vi "Torque_Application_11.20.vi"() -> ()   [LabVIEW 2016]
uses:
  Desktop/Controls_Framework_Spring17_LV14_pwm_1_enc_2(1)/Controls_Framework_Spring17_LV14_pwm_1_enc_2/Controls_Framework_Spring17_LV14_pwm_1_enc_2/FGVsandTypeDefs/System Selection.ctl
  Desktop/Controls_Framework_Spring17_LV14_pwm_1_enc_2(1)/Controls_Framework_Spring17_LV14_pwm_1_enc_2/Controls_Framework_Spring17_LV14_pwm_1_enc_2/FGVsandTypeDefs/Data Out.ctl
  Desktop/Controls_Framework_Spring17_LV14_pwm_1_enc_2(1)/Controls_Framework_Spring17_LV14_pwm_1_enc_2/Controls_Framework_Spring17_LV14_pwm_1_enc_2/tools/digitalArrayTool.vi
  Desktop/Controls_Framework_Spring17_LV14_pwm_1_enc_2(1)/Controls_Framework_Spring17_LV14_pwm_1_enc_2/Controls_Framework_Spring17_LV14_pwm_1_enc_2/hardware/ootb/OOTB Write.vi
  Desktop/Controls_Framework_Spring17_LV14_pwm_1_enc_2(1)/Controls_Framework_Spring17_LV14_pwm_1_enc_2/Controls_Framework_Spring17_LV14_pwm_1_enc_2/hardware/sadi/SADI Write.vi
  Desktop/Controls_Framework_Spring17_LV14_pwm_1_enc_2(1)/Controls_Framework_Spring17_LV14_pwm_1_enc_2/Controls_Framework_Spring17_LV14_pwm_1_enc_2/FGVsandTypeDefs/FGV System.vi
  <vilib>/Utility/semaphor.llb/Acquire Semaphore.vi
  Desktop/Controls_Framework_Spring17_LV14_pwm_1_enc_2(1)/Controls_Framework_Spring17_LV14_pwm_1_enc_2/Controls_Framework_Spring17_LV14_pwm_1_enc_2/hardware/simulations/MotorSimulation/SingleMotorSystem-HbridgeSimple-DAQ.vi
  Desktop/Controls_Framework_Spring17_LV14_pwm_1_enc_2(1)/Controls_Framework_Spring17_LV14_pwm_1_enc_2/Controls_Framework_Spring17_LV14_pwm_1_enc_2/hardware/simulations/MotorSimulation/DoubleMotorSystem-HbridgeTurnOn-DAQ.vi
  Desktop/Controls_Framework_Spring17_LV14_pwm_1_enc_2(1)/Controls_Framework_Spring17_LV14_pwm_1_enc_2/Controls_Framework_Spring17_LV14_pwm_1_enc_2/hardware/simulations/FurutaPendulum/FurutaPendulumSystem-HbridgeSimple-DAQ.vi
  <vilib>/Utility/semaphor.llb/Release Semaphore.vi
  Desktop/Controls_Framework_Spring17_LV14_pwm_1_enc_2(1)/Controls_Framework_Spring17_LV14_pwm_1_enc_2/Controls_Framework_Spring17_LV14_pwm_1_enc_2/hardware/ootb/OOTB Slowdown.vi
  Desktop/Controls_Framework_Spring17_LV14_pwm_1_enc_2(1)/Controls_Framework_Spring17_LV14_pwm_1_enc_2/Controls_Framework_Spring17_LV14_pwm_1_enc_2/hardware/ootb/OOTB Stop.vi
  Desktop/Controls_Framework_Spring17_LV14_pwm_1_enc_2(1)/Controls_Framework_Spring17_LV14_pwm_1_enc_2/Controls_Framework_Spring17_LV14_pwm_1_enc_2/hardware/sadi/SADI Slowdown.vi
  Desktop/Controls_Framework_Spring17_LV14_pwm_1_enc_2(1)/Controls_Framework_Spring17_LV14_pwm_1_enc_2/Controls_Framework_Spring17_LV14_pwm_1_enc_2/hardware/sadi/SADI Stop.vi
  <vilib>/Utility/semaphor.llb/Release Semaphore Reference.vi
panel:
  out "Numeric 3":i32=10818974
  out "AI0 3":dbl=2.506715973370057
  out "Torque End 2":dbl=964.1691552387538
  in  "+ Torque":dbl=100.0 format="%#_13g"
  in  "- Torque":dbl=-100.0 format="%#_13g"
  out "Torque 3":dbl=964.1691552387538
  out "AI Graph 3":dbl(graph)
  out "Torque 2":dbl=1035.2691658522822
  out "AI Graph 2":dbl(graph)
  out "Torque 1":dbl=964.1691552387538
  out "AI Graph 1":dbl(graph)
  out "Numeric":i32=10818974
  out "AI0":dbl=2.506715973370057
  out "Torque Before":dbl=964.1691552387538
  out "savedSections 2":u32 caption="# Sections Saved"
  out "saveTime 2":dbl caption="Total Save Time (s)" format="%#.3g"
  in  "Stop?":bool
  in  "Save?":bool
  in  "System":T1=enum."SADI DAQ"
  in  "Controller?":bool
  in  "AO Voltages [V]":cluster{"AO0":dbl, "AO1":dbl} {"AO1" min=0.0 max=5.0 step=0.01; "AO0" min=0.0 max=5.0 step=0.01}
  out "AI Voltages [V]":T2={"AI0"=2.4857487004494705, "AI1"=0.0018539516886717992, "AI2"=-0.01062114806262072, "AI3"=0.020274310509003104, "ENC0"=0, "ENC1"=0}
  in  "Tab Control":T3(tab)
  out "AI Graph":T4(graph)={"AI0"=2.4857487004494705, "AI1"=0.0018539516886717992, "AI2"=-0.01062114806262072, "AI3"=0.020274310509003104, "ENC0"=0, "ENC1"=0}
  # "Many of these controls are locked. Do not copy them.\nPlace a new control by right clicking anywhere in the front panel."
  # "v4.3.1"
  # "Time Information"
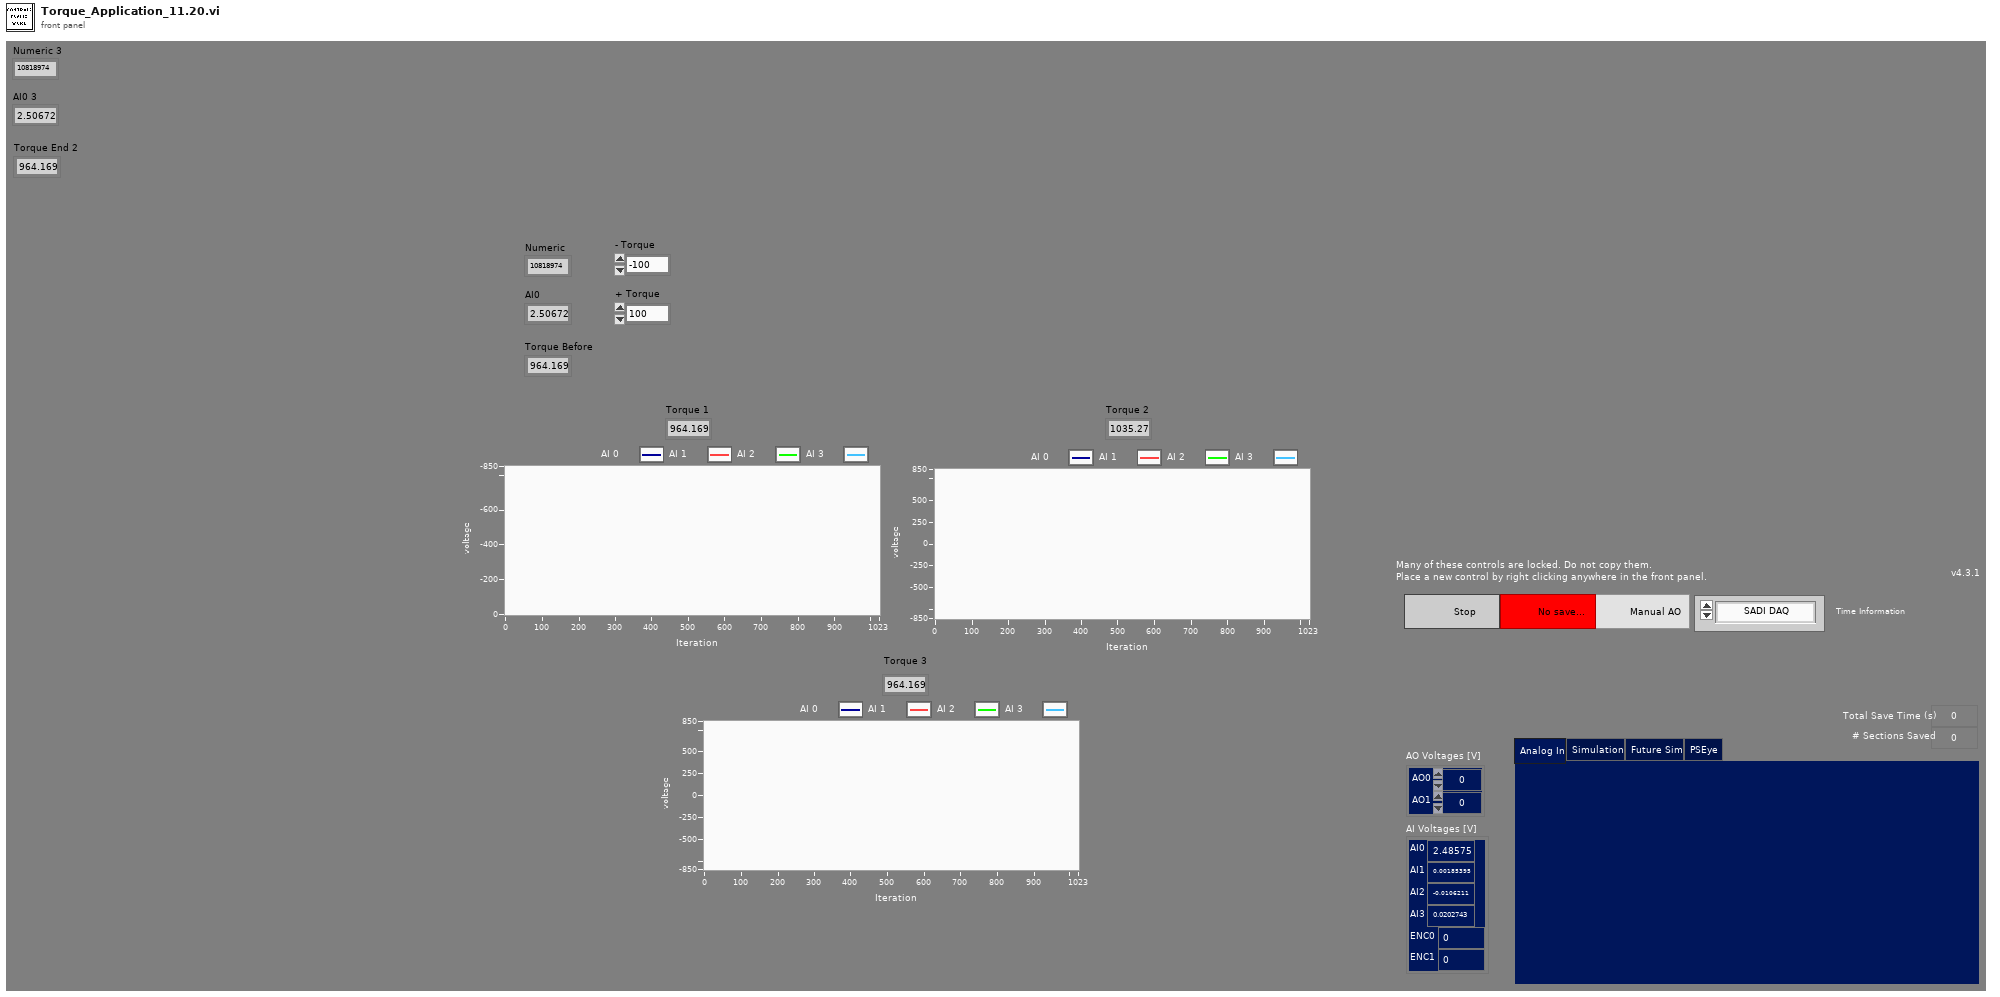
[diagram p1: front panel]
types:
  T1 = typedef "System Selection.ctl" = enum16{"OOTB DAQ", "SADI DAQ", "Single Motor Simulation", "Double Motor Simulation", "Furuta Pendulum"}
  T2 = typedef "Data Out.ctl" = cluster{"AI0":dbl, "AI1":dbl, "AI2":dbl, "AI3":dbl, "ENC0":i32, "ENC1":i32}
  T3 = enum32{"Analog In", "Simulation", "Future Sim", "PSEye"}
  T4 = cluster{"AI0":dbl, "AI1":dbl, "AI2":dbl, "AI3":dbl, "ENC0":i32, "ENC1":i32}
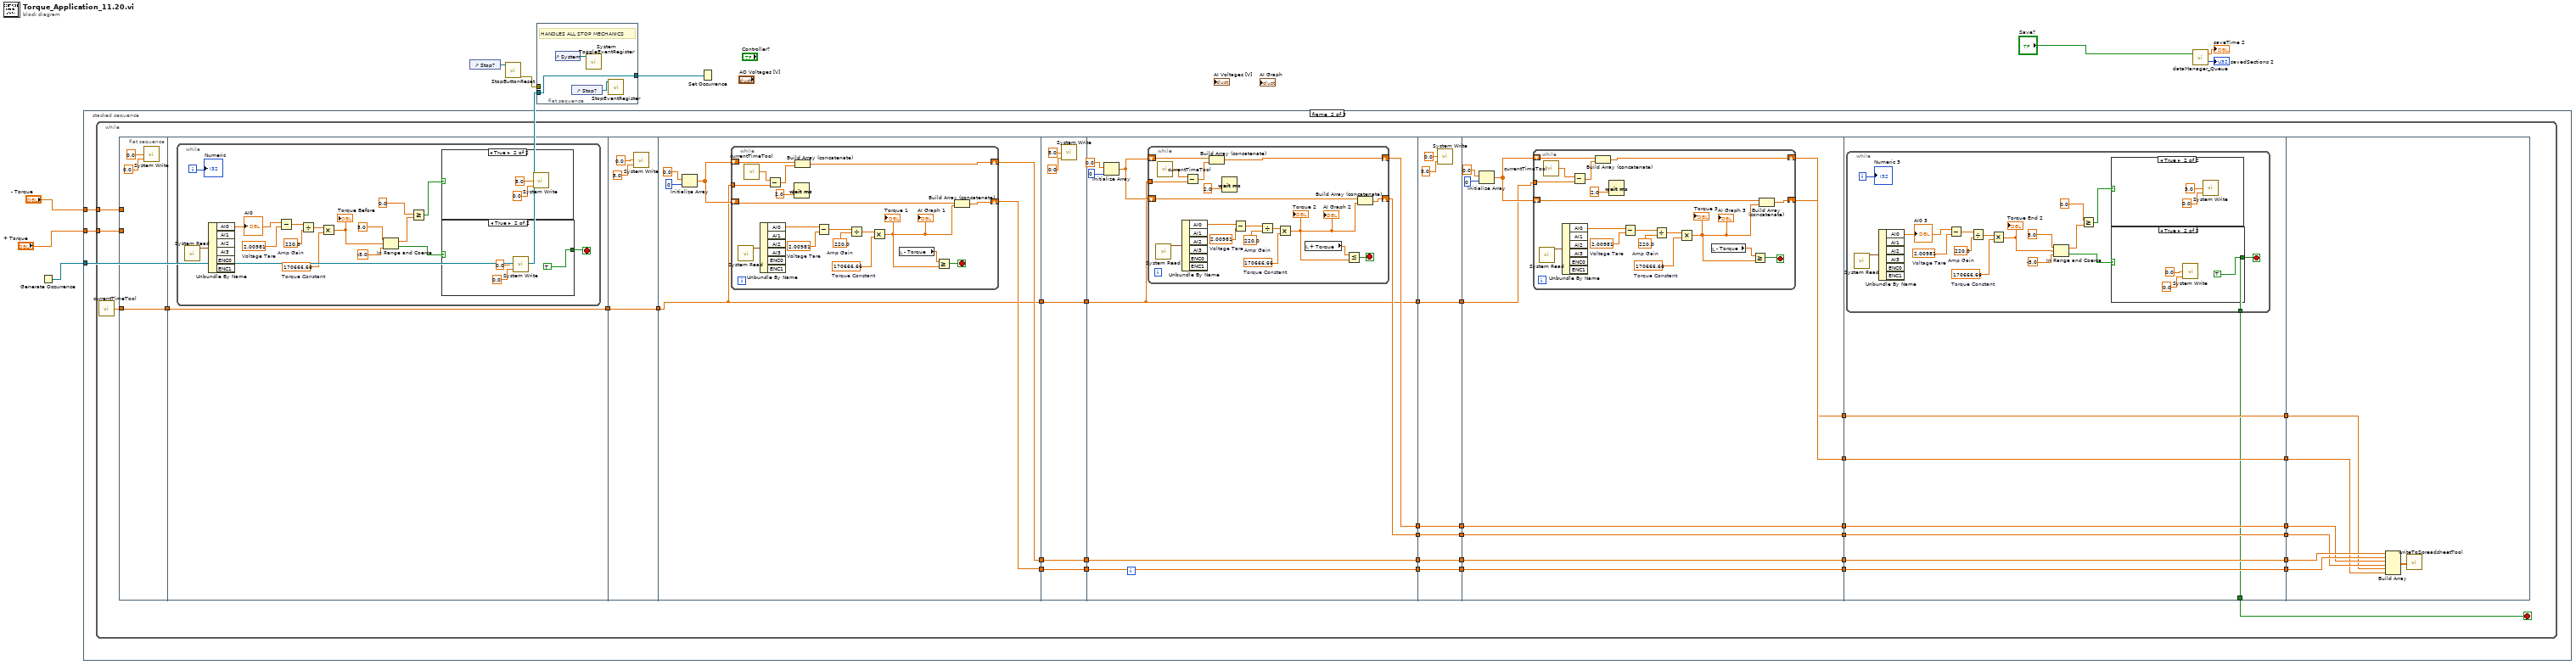
[diagram p0: block diagram]
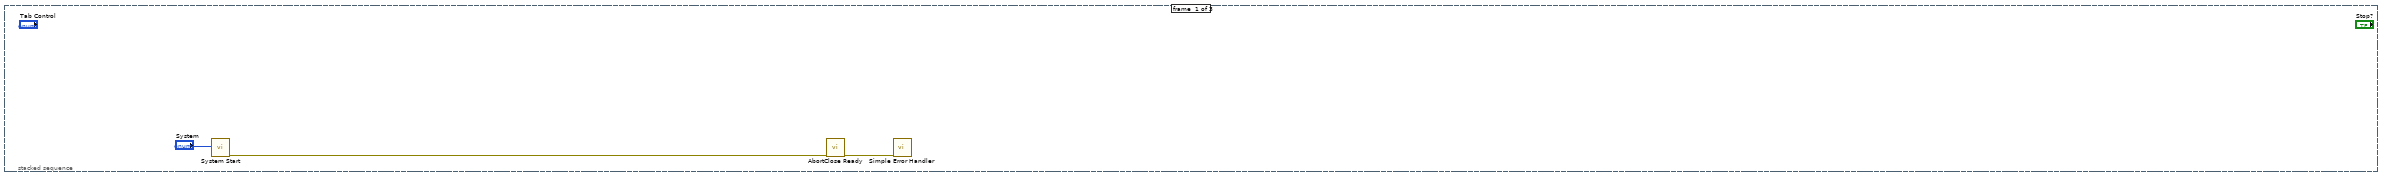
[diagram p2: hidden frame]
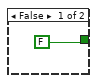
[diagram p3: hidden frame]
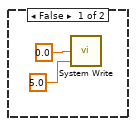
[diagram p4: hidden frame]
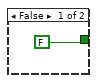
[diagram p5: hidden frame]
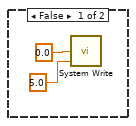
[diagram p6: hidden frame]
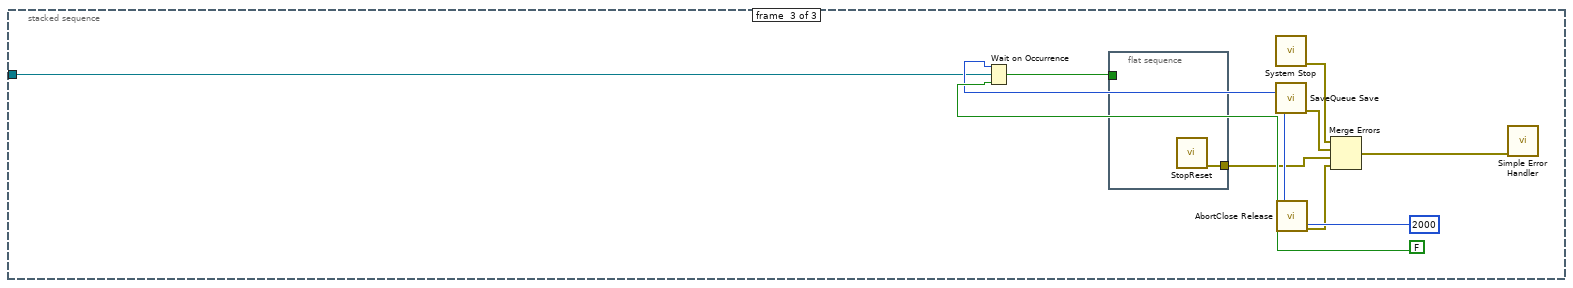
[diagram p7: hidden frame]
diagram:
  n1 = Generate Occurrence() -> (w7:refnum<k4>)
  n2 = stacked-sequence {
    tunnel: w7 -> [_ _ w212]
    tunnel: "- Torque" -> [_ w14 _]
    tunnel: "+ Torque" -> [_ w13 _]
    frame #0 {
      n3 = call "System Start.vi"("System"="System") -> ("error out"=w10:errorcluster)  [unwired: 9 in, 1 out]
      n4 = call "AbortClose Ready.vi"("error in (no error)"=w10) -> ("error out"=w11:errorcluster)  [unwired: 10 in]
      n5 = call <vilib>:"Simple Error Handler.vi"("error in (no error)"=w11) -> ()  [unwired: 4 in, 5 out]
    }
    frame #1 {
      n6 = while {
        tunnel: w14 -> [w49]
        tunnel: w13 -> [w48]
        stop <- w23 stop-if-true
        n7 = call "currentTimeTool.vi"() -> ("current time in seconds"=w19:dbl)
        n8 = flat-sequence {
          tunnel: w49 -> [_]
          tunnel: w48 -> [_]
          tunnel: [w50] -> w20
          tunnel: w19 -> [w50]
          tunnel: [w53] -> w21
          tunnel: w20 -> [w53]
          tunnel: [w78] -> w22
          tunnel: w21 -> [w78]
          tunnel: [w83] -> w44
          tunnel: [w82] -> w40
          tunnel: w22 -> [w81]
          tunnel: [w81] -> w17
          tunnel: [w107] -> w45
          tunnel: w44 -> [w107]
          tunnel: [w106] -> w41
          tunnel: w40 -> [w106]
          tunnel: [w105] -> w18
          tunnel: w17 -> [w105]
          tunnel: [w114] -> w46
          tunnel: w45 -> [w114]
          tunnel: [w113] -> w42
          tunnel: w41 -> [w113]
          tunnel: [w112] -> w38
          tunnel: [w111] -> w36
          tunnel: w18 -> [w110]
          tunnel: [w110] -> w15
          tunnel: [w140] -> w47
          tunnel: w46 -> [w140]
          tunnel: [w139] -> w43
          tunnel: w42 -> [w139]
          tunnel: [w138] -> w39
          tunnel: w38 -> [w138]
          tunnel: [w137] -> w37
          tunnel: w36 -> [w137]
          tunnel: [w136] -> w16
          tunnel: w15 -> [w136]
          tunnel: [w149] -> w35
          tunnel: w47 -> [w149]
          tunnel: [w148] -> w33
          tunnel: w43 -> [w148]
          tunnel: [w147] -> w31
          tunnel: w39 -> [w147]
          tunnel: [w146] -> w29
          tunnel: w37 -> [w146]
          tunnel: [w145] -> w27
          tunnel: [w144] -> w25
          tunnel: w16 -> [w143]
          tunnel: w35 -> [w177]
          tunnel: [w177] -> w34
          tunnel: w33 -> [w176]
          tunnel: [w176] -> w32
          tunnel: w31 -> [w175]
          tunnel: [w175] -> w30
          tunnel: w29 -> [w174]
          tunnel: [w174] -> w28
          tunnel: w27 -> [w173]
          tunnel: [w173] -> w26
          tunnel: w25 -> [w172]
          tunnel: [w172] -> w24
          tunnel: [w171] -> w23
          tunnel: w34 -> [w207]
          tunnel: w32 -> [w208]
          tunnel: w30 -> [w205]
          tunnel: w28 -> [w206]
          tunnel: w26 -> [w203]
          tunnel: w24 -> [w204]
          frame #0 {
            n9 = call "System Write.vi"("AO0"=0.0, "AO1"=0.0 ("AO0")) -> ()  [unwired: 6 in]
          }
          frame #1 {
            n10 = while {
              i -> [w69]
              stop <- w58 stop-if-true
              w55 = 170666.66  # Torque Constant
              w56 = 2.00981  # Voltage Tare
              w67 = 220.0  # Amp Gain
              n11 = call "System Read.vi"() -> ("Analog In and Encoders"=w68:T2)  [unwired: 5 in, 2 out]
              n12 = Unbundle By Name(w68) -> ("AI0"=w64:dbl)  [unwired: 5 out]
              "AI0" <- w64
              n13 = Subtract(x=w64, y=w56) -> (x-y=w65:dbl)
              n14 = Divide(x=w65, y=w67) -> (x/y=w66:dbl)
              n15 = Multiply(x=w66, y=w55) -> (x*y=w60:dbl)
              "Torque Before" <- w60
              n16 = In Range and Coerce(upper limit=5.0, x=w60, lower limit=-5.0) -> (coerced(x)=w59:dbl, In Range?=w57:bool)
              n17 = Greater Or Equal?(x=0.0, y=w59) -> (x >= y?=w61:bool)
              n18 = case shown="True" w61 {
                frame False {
                  n19 = call "System Write.vi"("AO0"=0.0, "AO1"=5.0 ("AO0")) -> ()  [unwired: 6 in]
                }
                frame True {
                  n20 = call "System Write.vi"("AO0"=5.0, "AO1"=0.0 ("AO0")) -> ()  [unwired: 6 in]
                }
              }
              n21 = case shown="True" w57 {
                tunnel: [FALSE TRUE] -> w58
                frame False {
                }
                frame True {
                  n22 = call "System Write.vi"("AO0"=0.0, "AO1"=0.0 ("AO0")) -> ()  [unwired: 6 in]
                }
              }
              "Numeric" <- w69
            }
          }
          frame #2 {
            n23 = call "System Write.vi"("AO0"=0.0, "AO1"=5.0 ("AO0")) -> ()  [unwired: 6 in]
          }
          frame #3 {
            n24 = Initialize Array(0.0, 0) -> (w84:dbl[])
            n25 = while {
              shift-right: [w98] -> w83
              shift-left: w84 -> [w97]
              shift-right: [w92] -> w82
              shift-left: w84 -> [w94]
              tunnel: w81 -> [w95]
              stop <- w99 stop-if-true
              w88 = 170666.66  # Torque Constant
              w89 = 2.00981  # Voltage Tare
              w103 = 220.0  # Amp Gain
              n26 = call "System Read.vi"() -> ("Analog In and Encoders"=w104:T2)  [unwired: 5 in, 2 out]
              n27 = call "currentTimeTool.vi"() -> ("current time in seconds"=w96:dbl)
              n28 = Unbundle By Name(w104) -> ("AI0"=w101:dbl)  [unwired: 5 out]
              n29 = Subtract(x=w96, y=w95) -> (x-y=w93:dbl)
              n30 = Wait (ms)(milliseconds to wait=2.0) -> ()  [unwired: 1 out]
              n31 = Build Array (concatenate)(w94, w93) -> (w92:dbl[])
              n32 = Subtract(x=w101, y=w89) -> (x-y=w100:dbl)
              n33 = Divide(x=w100, y=w103) -> (x/y=w102:dbl)
              n34 = Multiply(x=w102, y=w88) -> (x*y=w90:dbl)
              "Torque 1" <- w90
              "AI Graph 1" <- w90
              n35 = local read "- Torque"() -> (w91:dbl)
              n36 = Greater Or Equal?(x=w91, y=w90) -> (x >= y?=w99:bool)
              n37 = Build Array (concatenate)(w97, w90) -> (w98:dbl[])
            }
          }
          frame #4 {
            n38 = call "System Write.vi"("AO0"=5.0, "AO1"=0.0 ("AO0")) -> ()  [unwired: 6 in]
          }
          frame #5 {
            n39 = Initialize Array(0.0, 0) -> (w115:dbl[])
            n40 = while {
              shift-right: [w127] -> w112
              shift-left: w115 -> [w129]
              tunnel: w110 -> [w123]
              shift-right: [w122] -> w111
              shift-left: w115 -> [w124]
              stop <- w133 stop-if-true
              w119 = 170666.66  # Torque Constant
              w120 = 2.00981  # Voltage Tare
              w135 = 220.0  # Amp Gain
              n41 = call "System Read.vi"() -> ("Analog In and Encoders"=w132:T2)  [unwired: 5 in, 2 out]
              n42 = call "currentTimeTool.vi"() -> ("current time in seconds"=w125:dbl)
              n43 = Unbundle By Name(w132) -> ("AI0"=w131:dbl)  [unwired: 5 out]
              n44 = Subtract(x=w125, y=w123) -> (x-y=w126:dbl)
              n45 = Build Array (concatenate)(w124, w126) -> (w122:dbl[])
              n46 = Wait (ms)(milliseconds to wait=2.0) -> ()  [unwired: 1 out]
              n47 = Subtract(x=w131, y=w120) -> (x-y=w130:dbl)
              n48 = Divide(x=w130, y=w135) -> (x/y=w134:dbl)
              n49 = Multiply(x=w134, y=w119) -> (x*y=w128:dbl)
              "Torque 2" <- w128
              "AI Graph 2" <- w128
              n50 = local read "+ Torque"() -> (w121:dbl)
              n51 = Less Or Equal?(x=w121, y=w128) -> (x <= y?=w133:bool)
              n52 = Build Array (concatenate)(w129, w128) -> (w127:dbl[])
            }
          }
          frame #6 {
            n53 = call "System Write.vi"("AO0"=0.0, "AO1"=5.0 ("AO0")) -> ()  [unwired: 6 in]
          }
          frame #7 {
            n54 = Initialize Array(0.0, 0) -> (w150:dbl[])
            n55 = while {
              shift-right: [w163] -> w145
              shift-left: w150 -> [w164]
              tunnel: w143 -> [w160]
              shift-right: [w158] -> w144
              shift-left: w150 -> [w159]
              stop <- w165 stop-if-true
              w156 = 170666.66  # Torque Constant
              w157 = 2.00981  # Voltage Tare
              w169 = 220.0  # Amp Gain
              n56 = call "System Read.vi"() -> ("Analog In and Encoders"=w170:T2)  [unwired: 5 in, 2 out]
              n57 = call "currentTimeTool.vi"() -> ("current time in seconds"=w162:dbl)
              n58 = Unbundle By Name(w170) -> ("AI0"=w167:dbl)  [unwired: 5 out]
              n59 = Subtract(x=w162, y=w160) -> (x-y=w161:dbl)
              n60 = Build Array (concatenate)(w159, w161) -> (w158:dbl[])
              n61 = Wait (ms)(milliseconds to wait=2.0) -> ()  [unwired: 1 out]
              n62 = Subtract(x=w167, y=w157) -> (x-y=w166:dbl)
              n63 = Divide(x=w166, y=w169) -> (x/y=w168:dbl)
              n64 = Multiply(x=w168, y=w156) -> (x*y=w155:dbl)
              "Torque 3" <- w155
              "AI Graph 3" <- w155
              n65 = local read "- Torque"() -> (w154:dbl)
              n66 = Greater Or Equal?(x=w154, y=w155) -> (x >= y?=w165:bool)
              n67 = Build Array (concatenate)(w164, w155) -> (w163:dbl[])
            }
          }
          frame #8 {
            n68 = while {
              tunnel: [w179] -> w171
              i -> [w193]
              stop <- w179 stop-if-true
              w180 = 170666.66  # Torque Constant
              w181 = 2.00981  # Voltage Tare
              w191 = 220.0  # Amp Gain
              n69 = call "System Read.vi"() -> ("Analog In and Encoders"=w192:T2)  [unwired: 5 in, 2 out]
              n70 = Unbundle By Name(w192) -> ("AI0"=w188:dbl)  [unwired: 5 out]
              "AI0 3" <- w188
              n71 = Subtract(x=w188, y=w181) -> (x-y=w189:dbl)
              n72 = Divide(x=w189, y=w191) -> (x/y=w190:dbl)
              n73 = Multiply(x=w190, y=w180) -> (x*y=w184:dbl)
              "Torque End 2" <- w184
              n74 = In Range and Coerce(upper limit=5.0, x=w184, lower limit=-5.0) -> (coerced(x)=w183:dbl, In Range?=w182:bool)
              n75 = Greater Or Equal?(x=0.0, y=w183) -> (x >= y?=w185:bool)
              n76 = case shown="True" w185 {
                frame False {
                  n77 = call "System Write.vi"("AO0"=0.0, "AO1"=5.0 ("AO0")) -> ()  [unwired: 6 in]
                }
                frame True {
                  n78 = call "System Write.vi"("AO0"=5.0, "AO1"=0.0 ("AO0")) -> ()  [unwired: 6 in]
                }
              }
              n79 = case shown="True" w182 {
                tunnel: [FALSE TRUE] -> w179
                frame False {
                }
                frame True {
                  n80 = call "System Write.vi"("AO0"=0.0, "AO1"=0.0 ("AO0")) -> ()  [unwired: 6 in]
                }
              }
              "Numeric 3" <- w193
            }
          }
          frame #9 {
            n81 = Build Array(w208, w207, w206, w205, w204, w203) -> (w202:dbl[][])
            n82 = call "writeToSpreadsheetTool.vi"("2-d array of\nnumbers"=w202) -> ()
          }
        }
      }
    }
    frame #2 {
      n83 = Wait on Occurrence(1:FALSE ("ignore previous (T)"), 2:w212, 3:2000 ("ms timeout (-1)")) -> (0:w211:bool)
      n84 = flat-sequence {
        tunnel: w211 -> [_]
        tunnel: [w218] -> w210
        frame #0 {
          n85 = call "StopReset.vi"() -> ("error out"=w218:errorcluster)  [unwired: 11 in]
        }
      }
      n86 = call "System Stop.vi"() -> ("error out"=w216:errorcluster)  [unwired: 11 in]
      n87 = call "SaveQueue Save.vi"() -> ("error out"=w215:errorcluster)  [unwired: 11 in]
      n88 = call "AbortClose Release.vi"() -> ("error out"=w209:errorcluster)  [unwired: 11 in]
      n89 = Merge Errors(w216, w215, w210, w209) -> (w217:errorcluster)
      n90 = call <vilib>:"Simple Error Handler.vi"("error in (no error)"=w217) -> ()  [unwired: 1 in, 8 out]
    }
  }
  n91 = control-ref of="Stop?"() -> (w8:refnum<vi>)
  n92 = call "StopButtonReset.vi"("Boolean in"=w8) -> ("error out"=w9:errorcluster)  [unwired: 10 in]
  n93 = flat-sequence {
    tunnel: w9 -> [_]
    tunnel: w7 -> [w219]
    tunnel: [w219] -> w6
    frame #0 {
      # "HANDLES ALL STOP MECHANICS"
      n94 = control-ref of="System"() -> (w220:refnum<vi>)
      n95 = control-ref of="Stop?"() -> (w221:refnum<vi>)
      n96 = call "System ToggleEventRegister.vi"("System"=w220) -> ()  [unwired: 11 in]
      n97 = call "StopEventRegister.vi"("Stop Button Reference"=w221) -> ()  [unwired: 11 in]
    }
  }
  n98 = Set Occurrence(w6) -> ()
  n99 = call "dataManager_Queue.vi"("Save?"="Save?") -> ("savedSections 2"=→"savedSections 2":u32, "saveTime 2"=→"saveTime 2":dbl)  [unwired: 1 in]
